vi "update 用户最后动作.vi"(10 "用户名":string, 11 "数据库连接引用":T1) -> (0 "error out":errorcluster)   [LabVIEW 2013, in "数据库操作.lvclass"]
uses:
  <vilib>/addons/database/Connection.llb/Conn ObjectReference.ctl
  <vilib>/addons/database/Connection.llb/Conn Execute.vi
  <vilib>/addons/database/NI_Database_API.lvlib
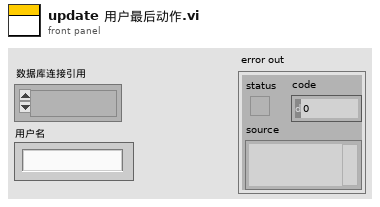
[diagram p1: front panel]
types:
  T1 = typedef "NI_Database_API.lvlib/Conn ObjectReference.ctl" = refnum<k1>
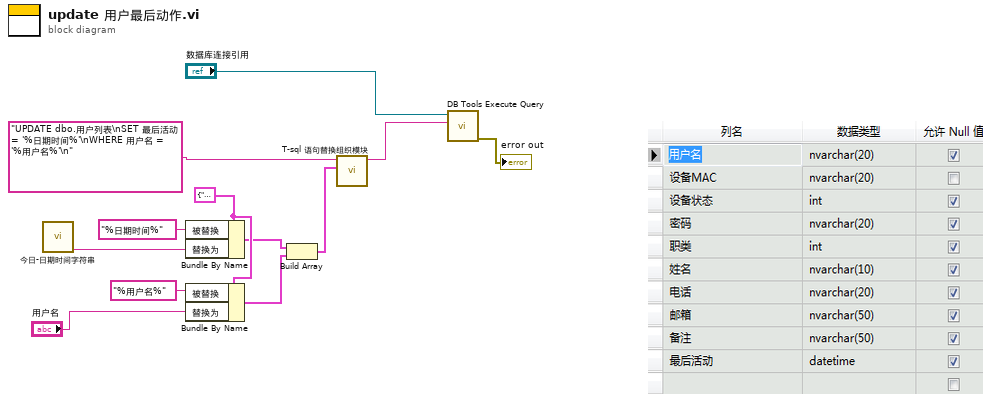
[diagram p0: block diagram]
diagram:
  w7 = cluster{"被替换":string, "替换为":string} {"被替换"="", "替换为"=""} ("替换单元")
  n1 = call "今日-日期时间字符串.vi"() -> ("日期时间"=w8:string)  [unwired: 9 in, 2 out]
  n2 = Bundle By Name(cluster=w7, "被替换"="%日期时间%", "替换为"=w8) -> (w6:cluster{"被替换":string, "替换为":string})
  n3 = Bundle By Name(cluster=w7, "被替换"="%用户名%", "替换为"="用户名") -> (w5:cluster{"被替换":string, "替换为":string})
  n4 = Build Array(w6, w5) -> (w3:cluster{"被替换":string, "替换为":string}[])
  n5 = call "T-sql 语句替换组织模块.vi"("替换项"=w3, "T-sql 模板"="UPDATE dbo.用户列表\nSET 最后活动 = '%日期时间%'\nWHERE 用户名 = '%用户名%'\n" ("SQL query")) -> ("T-sql"=w2:string)  [unwired: 8 in, 1 out]
  n6 = call-poly <vilib>:"DB Tools Execute Query.vi"("SQL query"=w2, "connection reference"="数据库连接引用") -> ("error out"=→"error out":errorcluster)  [unwired: 6 in, 1 out]
